vi "pallet labeling 2.vi"(0 "Array":dbl[][](array[numeric]), 1 "plt num":i32, 2 "curv num":i32) -> (14 "pallet situation":i16, 16 "camera pallet color":cluster{u32, u32}, 17 "ALARM":bool, 18 "sensor pallet color":cluster{u32, u32}, 19 "gb color":cluster{u32, u32})   [LabVIEW 2019]
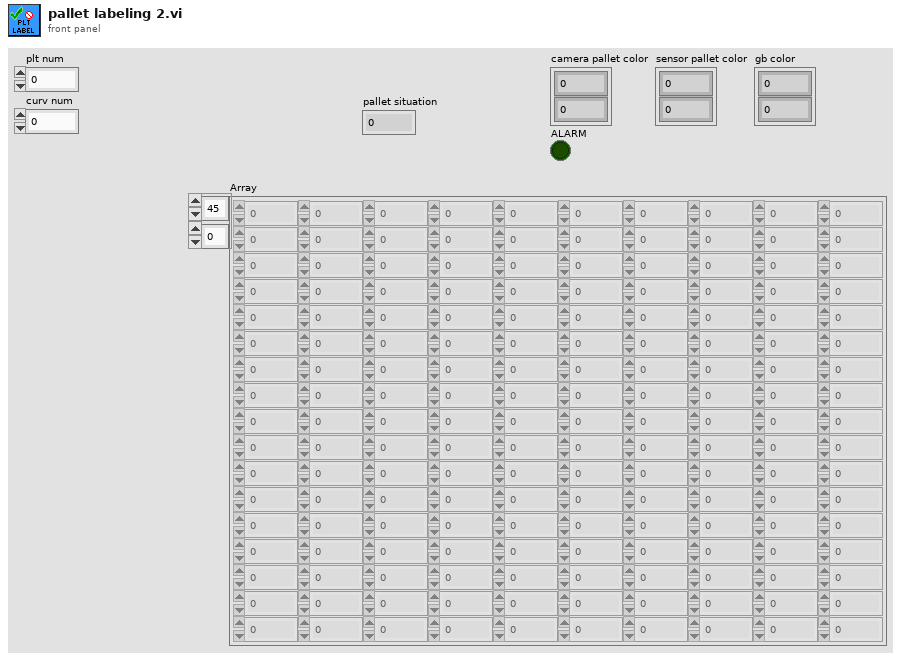
[diagram p1: front panel]
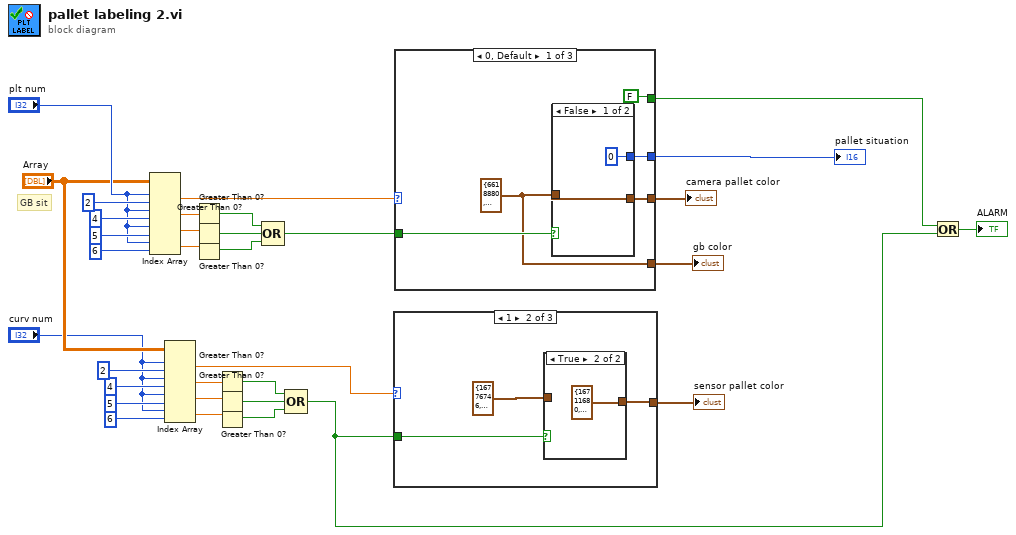
[diagram p0: block diagram]
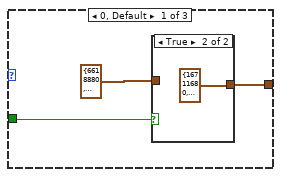
[diagram p2: hidden frame]
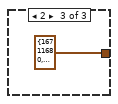
[diagram p5: hidden frame]
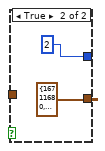
[diagram p6: hidden frame]
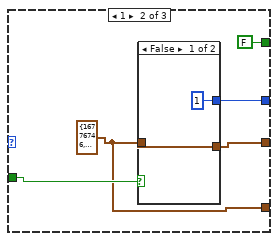
[diagram p7: hidden frame]
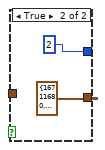
[diagram p8: hidden frame]
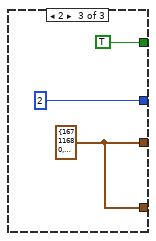
[diagram p9: hidden frame]
diagram:
  # "GB sit"
  n1 = Index Array(array="Array", index (row) #1="plt num", index (col) #1=2 ("disabled index (col)"), index (row) #2="plt num", index (col) #2=4 ("disabled index (col)"), index (row) #3="plt num", index (col) #3=5 ("disabled index (col)"), index (row) #4="plt num", index (col) #4=6 ("disabled index (col)")) -> (element #1=w32:dbl, element #2=w27:dbl, element #3=w28:dbl, element #4=w26:dbl)
  n2 = Index Array(array="Array", index (row) #1="curv num", index (col) #1=2 ("disabled index (col)"), index (row) #2="curv num", index (col) #2=4 ("disabled index (col)"), index (row) #3="curv num", index (col) #3=5 ("disabled index (col)"), index (row) #4="curv num", index (col) #4=6 ("disabled index (col)")) -> (element #1=w7:dbl, element #2=w10:dbl, element #3=w9:dbl, element #4=w8:dbl)
  n3 = Greater Than 0?(x=w27) -> (x > 0?=w25:bool)
  n4 = Greater Than 0?(x=w28) -> (x > 0?=w24:bool)
  n5 = Greater Than 0?(x=w26) -> (x > 0?=w23:bool)
  n6 = Greater Than 0?(x=w10) -> (x > 0?=w11:bool)
  n7 = Greater Than 0?(x=w9) -> (x > 0?=w12:bool)
  n8 = Greater Than 0?(x=w8) -> (x > 0?=w13:bool)
  n9 = Compound Arithmetic op=OR(w25, w24, w23) -> (w21:bool)
  n10 = Compound Arithmetic op=OR(w11, w12, w13) -> (w2:bool)
  n11 = case shown="1" w7 {
    tunnel: w2 -> [w35 w40 _]
    tunnel: [w34 w39 cluster{u32, u32} {16711680, 16711680} ("new element/subarray")] -> w6
    frame 0, Default {
      n12 = case shown="True" w35 {
        tunnel: [w37 cluster{u32, u32} {16711680, 16711680} ("new element/subarray")] -> w34
        tunnel: cluster{u32, u32} {6618880, 6618880} ("new element/subarray") -> [w37 _]
        frame False {
        }
        frame True {
        }
      }
    }
    frame 1 {
      n13 = case shown="True" w40 {
        tunnel: [w42 cluster{u32, u32} {16711680, 16711680} ("new element/subarray")] -> w39
        tunnel: cluster{u32, u32} {16776746, 16776746} ("new element/subarray") -> [w42 _]
        frame False {
        }
        frame True {
        }
      }
    }
    frame 2 {
    }
  }
  "sensor pallet color" <- w6
  n14 = case shown="0, Default" w32 {
    tunnel: w21 -> [w49 w57 _]
    tunnel: [w48 w58 w65] -> w22
    tunnel: [w47 w56 w65] -> w5
    tunnel: [w46 w55 2] -> w4
    tunnel: [FALSE FALSE TRUE] -> w3
    frame 0, Default {
      w47 = cluster{u32, u32} {6618880, 6618880} ("new element/subarray")
      n15 = case shown="False" w49 {
        tunnel: [w51 cluster{u32, u32} {16711680, 16711680} ("new element/subarray")] -> w48
        tunnel: w47 -> [w51 _]
        tunnel: [0 2] -> w46
        frame False {
        }
        frame True {
        }
      }
    }
    frame 1 {
      w56 = cluster{u32, u32} {16776746, 16776746} ("new element/subarray")
      n16 = case shown="False" w57 {
        tunnel: [w60 cluster{u32, u32} {16711680, 16711680} ("new element/subarray")] -> w58
        tunnel: w56 -> [w60 _]
        tunnel: [1 2] -> w55
        frame False {
        }
        frame True {
        }
      }
    }
    frame 2 {
      w65 = cluster{u32, u32} {16711680, 16711680} ("new element/subarray")
    }
  }
  "camera pallet color" <- w22
  "gb color" <- w5
  "pallet situation" <- w4
  n17 = Or(x=w3, y=w2) -> (x .or. y?=→"ALARM":bool)
